vi "Start Fan.vi"(8 "error in (no error)":errorcluster, 10 "Fan Speed":dbl, 11 "Fan Controller Ref":refnum<data-value>) -> (0 "error out":errorcluster, 3 "Fan Controller Ref out":refnum<data-value>)   [LabVIEW 2019, in "Fan Controller Ref.lvclass"]
uses:
  <vilib>/gpm_packages/@cs/Car-wash/Source/Fan Controller Ref/Fan Controller Ref.lvclass
  <vilib>/gpm_packages/@cs/Car-wash/Source/iFan Controller/iFan Controller.lvclass
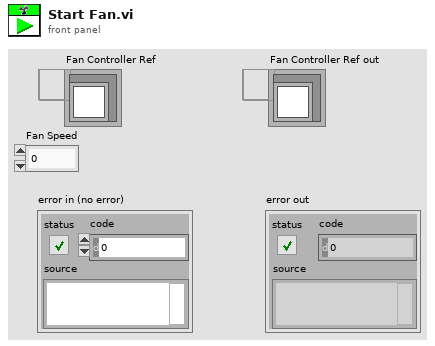
[diagram p1: front panel]
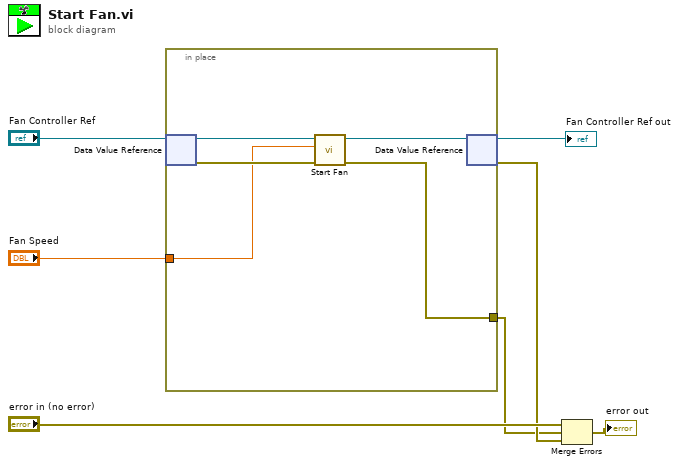
[diagram p0: block diagram]
diagram:
  n1 = in-place {
    in-place-border: "Fan Speed" -> [w9]
    in-place-border: [w8] -> w1
    n2 = in-place-dvr #1("Fan Controller Ref") -> (w12:refnum<class "iFan Controller.lvclass">, w10:errorcluster)
    n3 = call-dynamic "Start Fan.vi"("error in (no error)"=w10, "Fan Speed"=w9, "iFan Controller in"=w12) -> ("error out"=w8:errorcluster, "iFan Controller out"=w11:refnum<class "iFan Controller.lvclass">)  [unwired: 7 in]
    n4 = in-place-dvr #1(w11) -> (→"Fan Controller Ref out":refnum<data-value>, w2:errorcluster)
  }
  n5 = Merge Errors("error in (no error)", w1, w2) -> (→"error out":errorcluster)
